vi "Method.vi"(8 "error in (no error)":errorcluster, 11 "Child 1 in":refnum<class "Child 1.lvclass">) -> (0 "error out":errorcluster, 2 "Output":string, 3 "Child 1 out":refnum<class "Child 1.lvclass">)   [LabVIEW 2017, in "Child 1.lvclass"]
uses:
  Child 1.lvclass
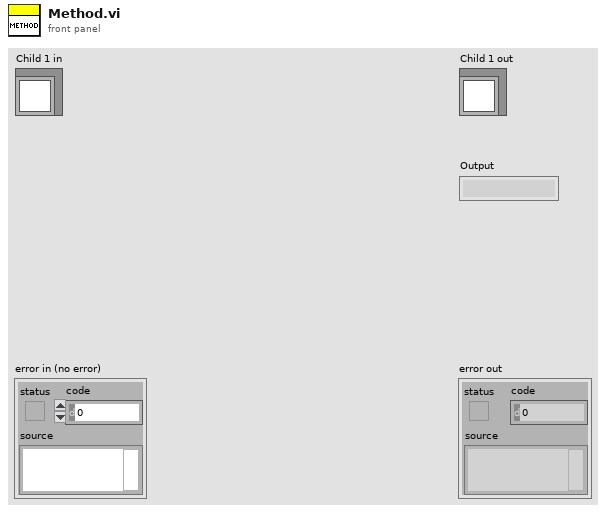
[diagram p1: front panel]
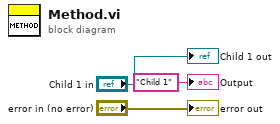
[diagram p0: block diagram]
diagram:
  "error out" <- "error in (no error)"
  "Child 1 out" <- "Child 1 in"
  "Output" <- "Child 1" ("Output")
